vi "change f values.vi"(6 "index (col)":i32, 7 "new element":dbl, 8 "frekans index":dbl, 9 "Frekanslar":dbl[](array[numeric]), 10 "F Values Array":dbl[][](array[numeric]), 11 "LstBox Refnum":refnum<vi>) -> (3 "output array":dbl[][](array[numeric]))   [LabVIEW 2014]
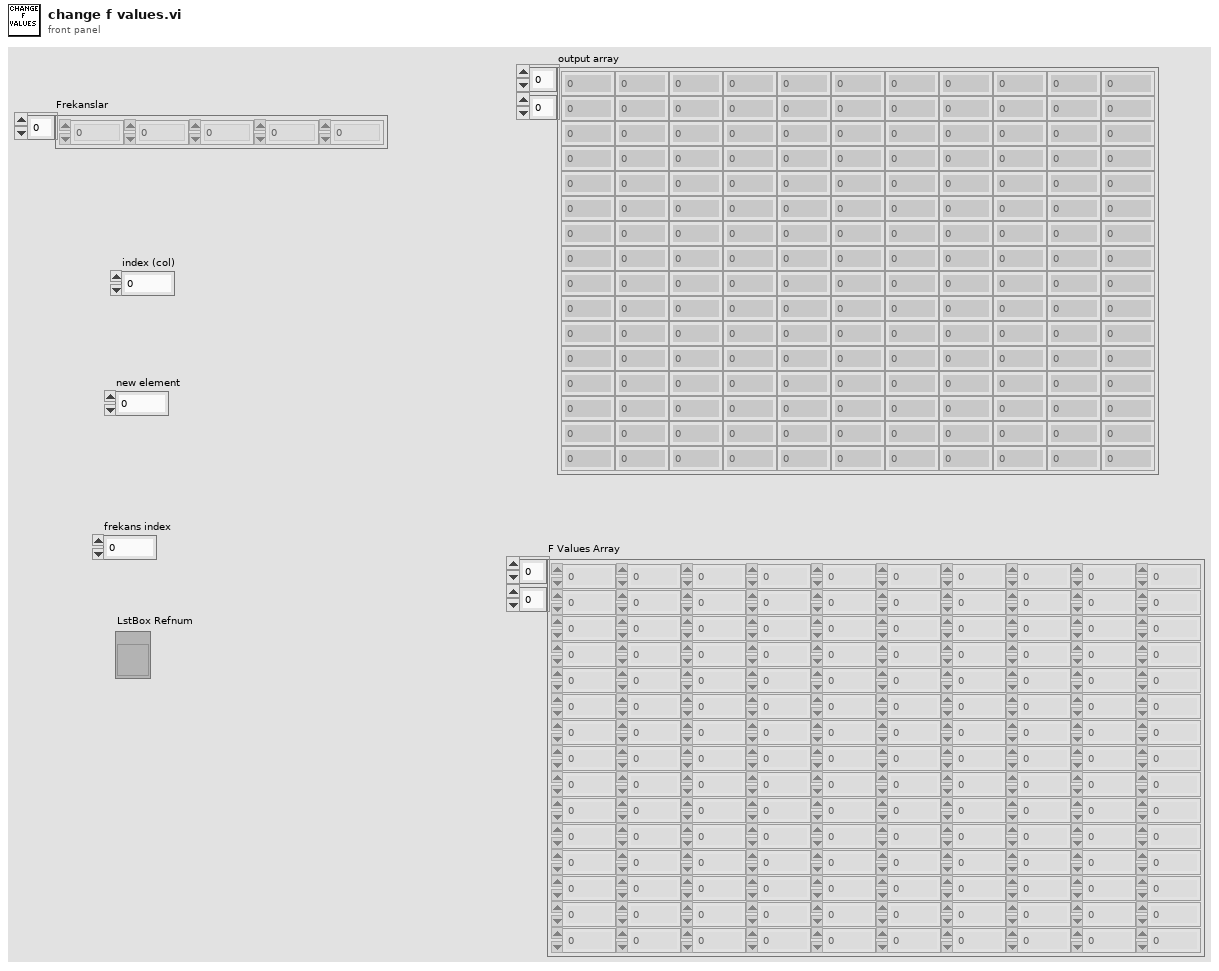
[diagram p1: front panel]
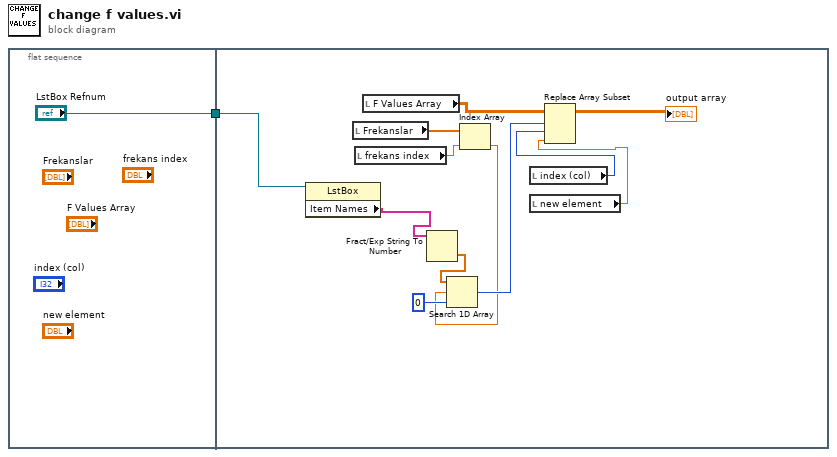
[diagram p0: block diagram]
diagram:
  n1 = flat-sequence {
    tunnel: ["LstBox Refnum"] -> w1
    tunnel: w1 -> [w7]
    frame #0 {
    }
    frame #1 {
      n2 = property class="LstBox"(reference=w7) -> ("Item Names"=w6:string[])  [unwired: 1 in, 2 out]
      n3 = local read "Frekanslar"() -> (w8:dbl[])
      n4 = local read "frekans index"() -> (w9:dbl)
      n5 = local read "F Values Array"() -> (w14:dbl[][])
      n6 = Fract/Exp String To Number(string=w6) -> (number=w11:dbl[])  [unwired: 3 in, 1 out]
      n7 = Index Array(array=w8, index=w9) -> (element=w10:dbl)
      n8 = Search 1D Array(1D array=w11, element=w10, start index (0)=0) -> (index of element=w13:i32)
      n9 = local read "index (col)"() -> (w5:i32)
      n10 = local read "new element"() -> (w4:dbl)
      n11 = Replace Array Subset(array=w14, new element=w4, index (row)=w13, index (col)=w5) -> (→"output array":dbl[][])
    }
  }
